vi "Output_opt.vi"(0 "Activation Function":enum32{"Sigmoid", "RELU", "Tanh", "Leaky RELU"}(ring), 1 "Activation l-1":dbl[](array[numeric]), 2 "Weights":dbl[](array[numeric]), 3 "Biases":dbl, 5 "Activation":dbl, 7 "Net Output":dbl, 9 "Target":dbl, 12 "Weight Regularizers":enum32{"None", "L1", "L2"}(radio), 13 "Adam Data In":T1) -> (4 "Delta":dbl, 6 "Updated Weights":dbl[](array[numeric]), 8 "Updated Biases":dbl, 14 "Adam Data Out":T1)   [LabVIEW 2018]
uses:
  Adam_data.ctl
  Globals.vi
  Iteration Counter.vi
panel:
  out "Grad. w":dbl[](array[numeric])
  out "Grad. b":dbl
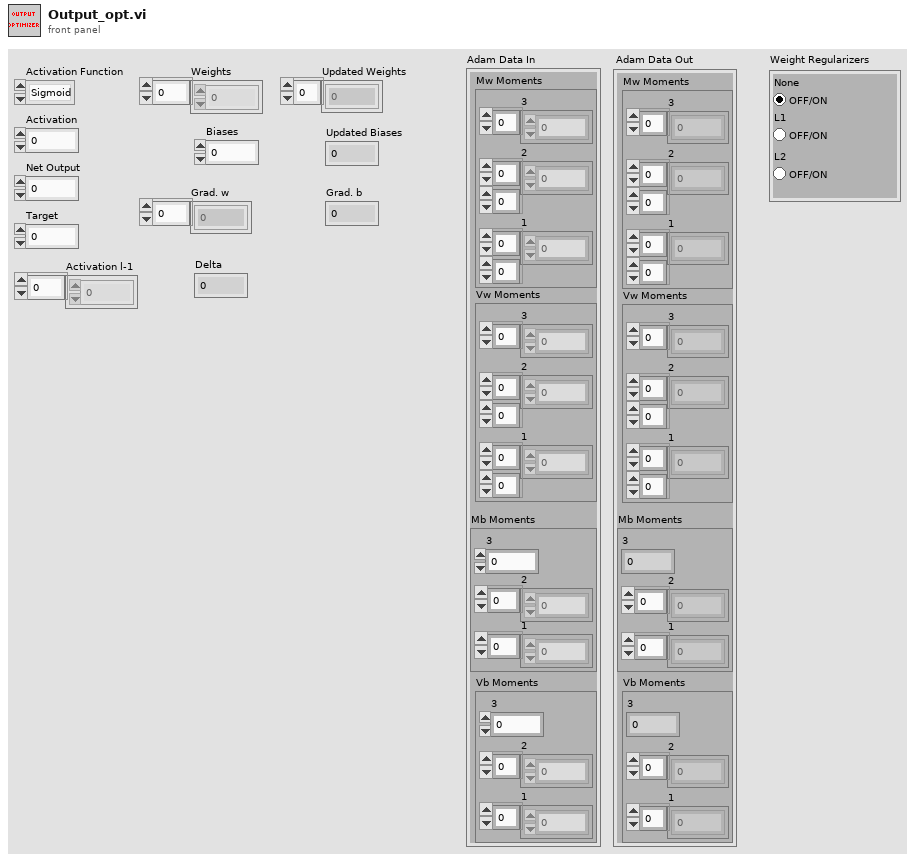
[diagram p1: front panel]
types:
  T1 = typedef "Adam_data.ctl" = cluster{"Mw Moments":cluster{"3 ":dbl[], "2":dbl[][], "1":dbl[][]}, "Vw Moments":cluster{"3":dbl[], "2":dbl[][], "1":dbl[][]}, "Mb Moments":cluster{"3":dbl, "2":dbl[], "1":dbl[]}, "Vb Moments":cluster{"3":dbl, "2":dbl[], "1":dbl[]}}
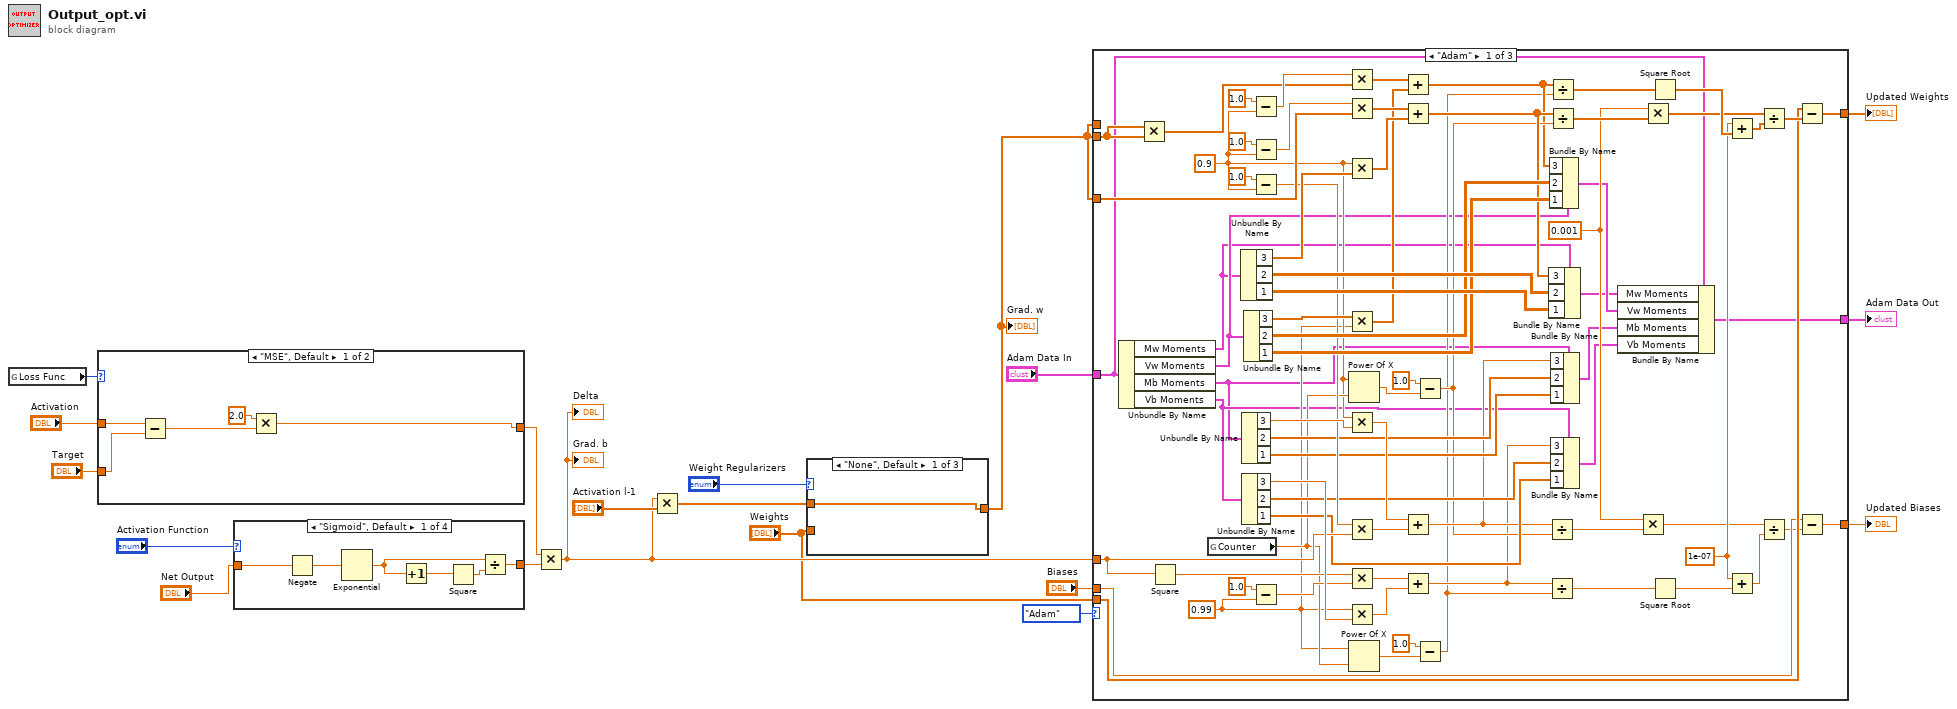
[diagram p0: block diagram]
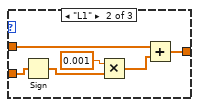
[diagram p2: hidden frame]
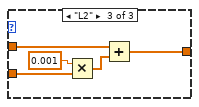
[diagram p3: hidden frame]
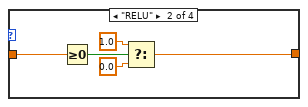
[diagram p6: hidden frame]
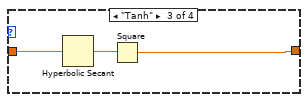
[diagram p7: hidden frame]
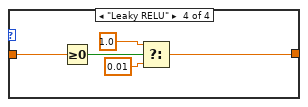
[diagram p8: hidden frame]
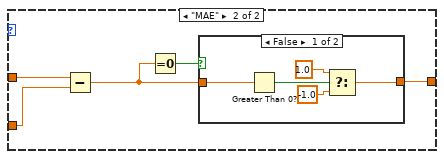
[diagram p9: hidden frame]
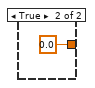
[diagram p10: hidden frame]
diagram:
  n1 = global read "Globals.vi" "Loss Func"() -> (w19:enum16{"MSE", "MAE"})
  n2 = case shown="\"MSE\", Default" w19 {
    tunnel: "Activation" -> [w23 w28]
    tunnel: "Target" -> [w22 w29]
    tunnel: [w20 w26] -> w15
    frame "MSE", Default {
      n3 = Subtract(x=w23, y=w22) -> (x-y=w21:dbl)
      n4 = Multiply(x=2.0, y=w21) -> (x*y=w20:dbl)
    }
    frame "MAE" {
      n5 = Subtract(x=w28, y=w29) -> (x-y=w25:dbl)
      n6 = Equal To 0?(x=w25) -> (x = 0?=w27:bool)
      n7 = case shown="False" w27 {
        tunnel: [w30 0.0] -> w26
        tunnel: w25 -> [w34 _]
        frame False {
          n8 = Greater Than 0?(x=w34) -> (x > 0?=w33:bool)
          n9 = Select(t=1.0, s=w33, f=-1.0) -> (s? t:f=w30:dbl)
        }
        frame True {
        }
      }
    }
  }
  n10 = case shown="\"Sigmoid\", Default" "Activation Function" {
    tunnel: "Net Output" -> [w37 w45 w48 w52]
    tunnel: [w36 w46 w47 w51] -> w14
    frame "Sigmoid", Default {
      n11 = Negate(x=w37) -> (-x=w41:dbl)
      n12 = Exponential(1:w41) -> (0:w38:dbl)
      n13 = Increment(x=w38) -> (x+1=w40:dbl)
      n14 = Square(x=w40) -> (x^2=w39:dbl)
      n15 = Divide(x=w38, y=w39) -> (x/y=w36:dbl)
    }
    frame "RELU" {
      n16 = Greater Or Equal To 0?(x=w45) -> (x >= 0?=w42:bool)
      n17 = Select(t=1.0, s=w42, f=0.0) -> (s? t:f=w46:dbl)
    }
    frame "Tanh" {
      n18 = Hyperbolic Secant(1:w48) -> (0:w49:dbl)
      n19 = Square(x=w49) -> (x^2=w47:dbl)
    }
    frame "Leaky RELU" {
      n20 = Greater Or Equal To 0?(x=w52) -> (x >= 0?=w50:bool)
      n21 = Select(t=1.0, s=w50, f=0.01) -> (s? t:f=w51:dbl)
    }
  }
  n22 = Multiply(x=w15, y=w14) -> (x*y=w11:dbl)
  "Delta" <- w11
  "Grad. b" <- w11
  n23 = Multiply(x=w11, y="Activation l-1") -> (x*y=w3:dbl[])
  n24 = case shown="\"None\", Default" "Weight Regularizers" {
    tunnel: w3 -> [w55 w57 w66]
    tunnel: [w55 w56 w62] -> w2
    tunnel: "Weights" -> [_ w60 w64]
    frame "None", Default {
    }
    frame "L1" {
      n25 = Sign(1:w60) -> (0:w59:dbl[])
      n26 = Multiply(x=0.001, y=w59) -> (x*y=w58:dbl[])
      n27 = Add(x=w57, y=w58) -> (x+y=w56:dbl[])
    }
    frame "L2" {
      n28 = Multiply(x=0.001, y=w64) -> (x*y=w63:dbl[])
      n29 = Add(x=w66, y=w63) -> (x+y=w62:dbl[])
    }
  }
  "Grad. w" <- w2
  n30 = case shown="\"Adam\"" enum16{"Adagrad", "Adadelta", "Adam"}."Adam" ("Optimizer") {
    tunnel: w2 -> [_ _ _]
    tunnel: w2 -> [w136 _ _]
    tunnel: w2 -> [w129 _ _]
    tunnel: w11 -> [w114 _ _]
    tunnel: "Weights" -> [w88 w143 w146]
    tunnel: [w87 w143 w146] -> w10
    tunnel: "Biases" -> [w79 w142 w145]
    tunnel: [w77 w142 w145] -> w8
    tunnel: "Adam Data In" -> [w72 w141 w144]
    tunnel: [w67 w141 w144] -> w6
    frame "Adam" {
      w84 = 1e-07
      w83 = 0.001
      w105 = 0.99
      w106 = 0.9
      n31 = Unbundle By Name(w72) -> ("Mw Moments"=w73:cluster{"3 ":dbl[], "2":dbl[][], "1":dbl[][]}, "Vw Moments"=w74:cluster{"3":dbl[], "2":dbl[][], "1":dbl[][]}, "Mb Moments"=w75:cluster{"3":dbl, "2":dbl[], "1":dbl[]}, "Vb Moments"=w76:cluster{"3":dbl, "2":dbl[], "1":dbl[]})
      n32 = Multiply(x=w129, y=w129) -> (x*y=w128:dbl[])
      n33 = Square(x=w114) -> (x^2=w112:dbl)
      n34 = global read "Iteration Counter.vi" "Counter"() -> (w107:dbl)
      n35 = Unbundle By Name(w73) -> ("3"=w140:dbl[], "2"=w134:dbl[][], "1"=w133:dbl[][])
      n36 = Unbundle By Name(w75) -> ("3"=w123:dbl, "2"=w118:dbl[], "1"=w117:dbl[])
      n37 = Unbundle By Name(w76) -> ("3"=w116:dbl, "2"=w109:dbl[], "1"=w108:dbl[])
      n38 = Unbundle By Name(w74) -> ("3"=w132:dbl[], "2"=w125:dbl[][], "1"=w124:dbl[][])
      n39 = Subtract(x=1.0, y=w106) -> (x-y=w130:dbl)
      n40 = Subtract(x=1.0, y=w106) -> (x-y=w137:dbl)
      n41 = Subtract(x=1.0, y=w106) -> (x-y=w121:dbl)
      n42 = Subtract(x=1.0, y=w105) -> (x-y=w113:dbl)
      n43 = Multiply(x=w130, y=w128) -> (x*y=w126:dbl[])
      n44 = Multiply(x=w137, y=w136) -> (x*y=w135:dbl[])
      n45 = Multiply(x=w106, y=w140) -> (x*y=w138:dbl[])
      n46 = Multiply(x=w132, y=w105) -> (x*y=w127:dbl[])
      n47 = Multiply(x=w106, y=w123) -> (x*y=w119:dbl)
      n48 = Multiply(x=w121, y=w114) -> (x*y=w120:dbl)
      n49 = Multiply(x=w112, y=w113) -> (x*y=w111:dbl)
      n50 = Multiply(x=w105, y=w116) -> (x*y=w110:dbl)
      n51 = Power Of X(1:w107, 2:w106) -> (0:w103:dbl)
      n52 = Power Of X(1:w107, 2:w105) -> (0:w101:dbl)
      n53 = Add(x=w126, y=w127) -> (x+y=w97:dbl[])
      n54 = Add(x=w135, y=w138) -> (x+y=w100:dbl[])
      n55 = Add(x=w119, y=w120) -> (x+y=w99:dbl)
      n56 = Add(x=w111, y=w110) -> (x+y=w96:dbl)
      n57 = Subtract(x=1.0, y=w103) -> (x-y=w98:dbl)
      n58 = Subtract(x=1.0, y=w101) -> (x-y=w95:dbl)
      n59 = Divide(x=w99, y=w98) -> (x/y=w82:dbl)
      n60 = Divide(x=w96, y=w95) -> (x/y=w86:dbl)
      n61 = Divide(x=w97, y=w95) -> (x/y=w94:dbl[])
      n62 = Divide(x=w100, y=w98) -> (x/y=w92:dbl[])
      n63 = Bundle By Name(cluster=w73, "3"=w100, "2"=w134, "1"=w133) -> (w68:cluster{"3 ":dbl[], "2":dbl[][], "1":dbl[][]})
      n64 = Bundle By Name(cluster=w74, "3"=w97, "2"=w125, "1"=w124) -> (w69:cluster{"3":dbl[], "2":dbl[][], "1":dbl[][]})
      n65 = Bundle By Name(cluster=w75, "3"=w99, "2"=w118, "1"=w117) -> (w70:cluster{"3":dbl, "2":dbl[], "1":dbl[]})
      n66 = Bundle By Name(cluster=w76, "3"=w96, "2"=w109, "1"=w108) -> (w71:cluster{"3":dbl, "2":dbl[], "1":dbl[]})
      n67 = Bundle By Name(cluster=w72, "Mw Moments"=w68, "Vw Moments"=w69, "Mb Moments"=w70, "Vb Moments"=w71) -> (w67:T1)
      n68 = Multiply(x=w83, y=w82) -> (x*y=w81:dbl)
      n69 = Multiply(x=w83, y=w92) -> (x*y=w91:dbl[])
      n70 = Square Root(x=w94) -> (sqrt(x)=w93:dbl[])
      n71 = Square Root(x=w86) -> (sqrt(x)=w85:dbl)
      n72 = Add(x=w84, y=w93) -> (x+y=w90:dbl[])
      n73 = Add(x=w84, y=w85) -> (x+y=w80:dbl)
      n74 = Divide(x=w91, y=w90) -> (x/y=w89:dbl[])
      n75 = Divide(x=w81, y=w80) -> (x/y=w78:dbl)
      n76 = Subtract(x=w88, y=w89) -> (x-y=w87:dbl[])
      n77 = Subtract(x=w79, y=w78) -> (x-y=w77:dbl)
    }
    frame "Adadelta" {
    }
    frame "Adagrad" {
    }
  }
  "Updated Weights" <- w10
  "Updated Biases" <- w8
  "Adam Data Out" <- w6
